vi "Set Bias Voltage.vi"(8 "error in (no error)":errorcluster, 9 "Channel":u32, 10 "Bias Voltage (V)":dbl, 11 "Instrument.VSource in":refnum<class "Instrument.VSource.lvclass">) -> (0 "error out":errorcluster, 3 "Instrument.VSource out":refnum<class "Instrument.VSource.lvclass">)   [LabVIEW 2019, in "Instrument.VSource.lvclass"]
uses:
  Instrument.VSource.lvclass
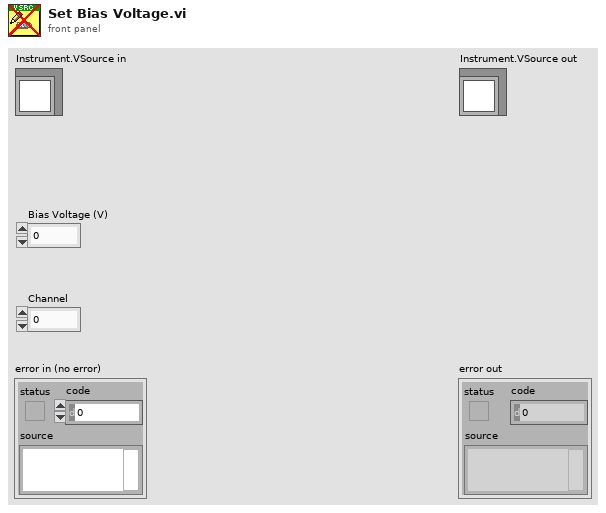
[diagram p1: front panel]
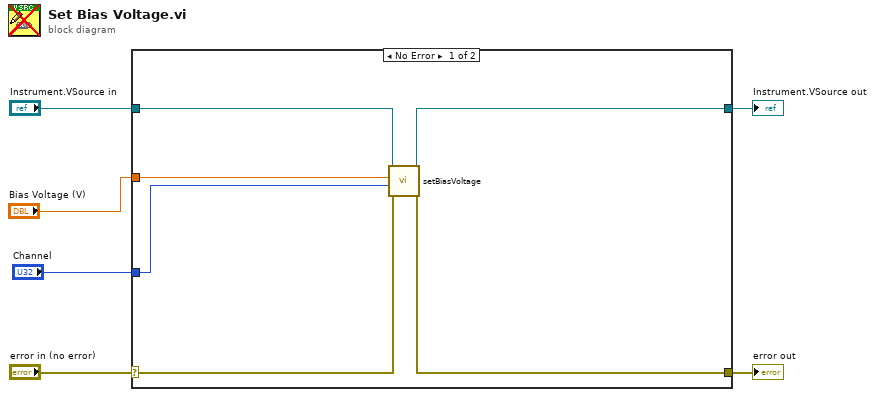
[diagram p0: block diagram]
diagram:
  n1 = case shown="No Error" "error in (no error)" {
    selector: "error in (no error)" -> [w9 w14]
    tunnel: [w8 w14] -> w5
    tunnel: [w11 w13] -> w3
    tunnel: "Instrument.VSource in" -> [w10 w13]
    tunnel: "Bias Voltage (V)" -> [w12 _]
    tunnel: "Channel" -> [w7 _]
    frame No Error {
      n2 = call-dynamic "setBiasVoltage.vi"("error in (no error)"=w9, "Channel"=w7, "Bias Voltage (V)"=w12, "Instrument.VSource in"=w10) -> ("error out"=w8:errorcluster, "Instrument.VSource out"=w11:refnum<class "Instrument.VSource.lvclass">)  [unwired: 6 in]
    }
    frame Error {
    }
  }
  "error out" <- w5
  "Instrument.VSource out" <- w3
